vi "Example XYGraph Set BGK Color.vi"() -> ()   [LabVIEW 2020]
uses:
  Graph Extensions.lvlib
panel:
  in  "Color Box":u32(colorbox)
  out "XY Graph":cluster{dbl[], dbl[]}[](graph)
  # "Set any color here, the \ngrid lines will automatically\nbe adjusted for easy viewing"
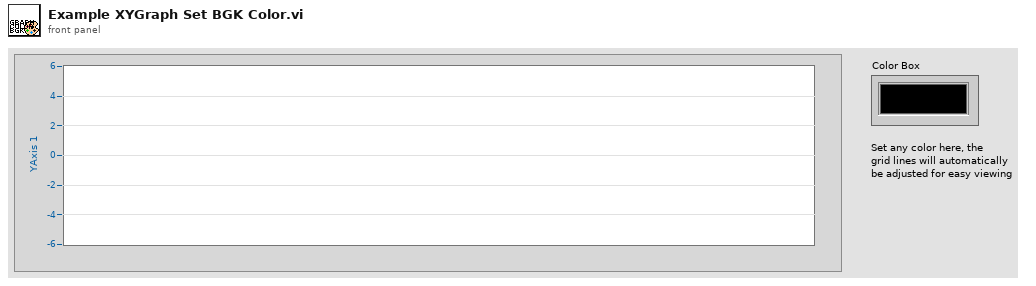
[diagram p1: front panel]
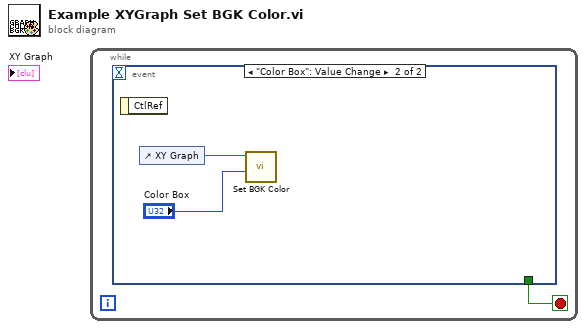
[diagram p0: block diagram]
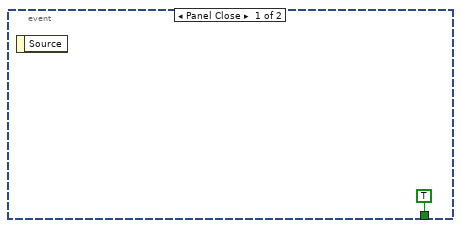
[diagram p2: hidden frame]
diagram:
  n1 = while {
    stop <- w1 stop-if-true
    n2 = event shown="[1] \"Color Box\": Value Change" {
      selector: _ -> [_ _]
      dyn-events: _ -> [_ _]
      timeout: _ -> [_ _]
      tunnel: [TRUE _] -> w1
      event Panel Close {
        n3 = event-data() -> ()  [unwired: 1 in, 1 out]
      }
      event "Color Box": Value Change {
        n4 = event-data() -> ()  [unwired: 1 in, 1 out]
        n5 = control-ref of="XY Graph"() -> (w3:refnum<vi>)
        n6 = call "Set BGK Color.vi"("color"="Color Box", "XYGraph"=w3) -> ()  [unwired: 8 in, 2 out]
      }
    }
  }
